vi "LWXPS_PositionerCompensationPreFeedForwardPhaseCorrectionFilterSet.vi"(0 "Positioner Name":string, 1 "XPS Reference IN":refnum<k24>, 5 "Filter Number":i32, 7 "Numerator Frequency":dbl, 9 "Denominator Frequency":dbl, 11 "Phase Correction Gain":dbl, 12 "LabVIEW error IN":errorcluster) -> (4 "XPS Reference OUT":refnum<k24>, 6 "Returned error code":i32, 8 "XPS Error String":string, 15 "LabVIEW error OUT":errorcluster)   [LabVIEW 2014]
uses:
  D:/XPSQ8_LabView_Library/Development/Source/Dll/Newport.XPS.CommandInterface.dll
  Dll/Newport.XPS.CommandInterface.dll
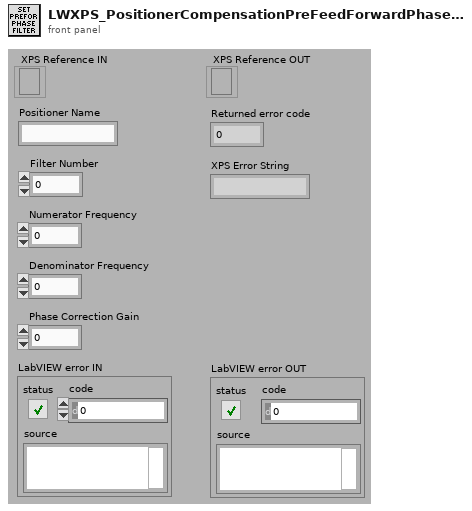
[diagram p1: front panel]
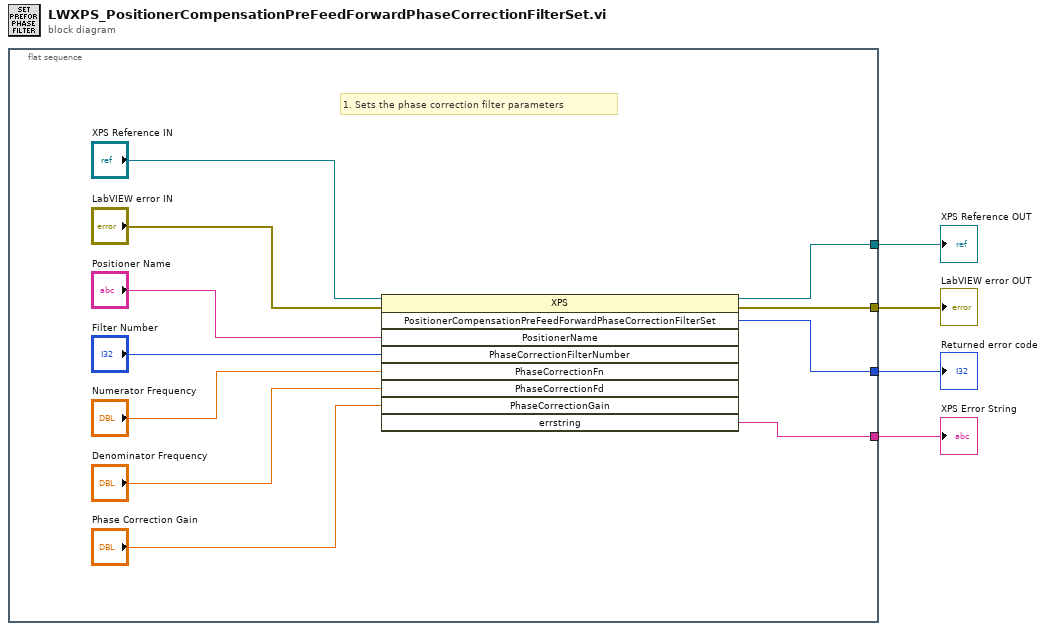
[diagram p0: block diagram]
diagram:
  n1 = flat-sequence {
    tunnel: [w11] -> w4
    tunnel: [w10] -> w3
    tunnel: [w12] -> w2
    tunnel: [w8] -> w1
    frame #0 {
      # "1. Sets the phase correction filter parameters"
      n2 = invoke class="XPS" method="PositionerCompensationPreFeedForwardPhaseCorrectionFilterSet"(reference="XPS Reference IN", error in="LabVIEW error IN", "PositionerName"="Positioner Name", "PhaseCorrectionFilterNumber"="Filter Number", "PhaseCorrectionFn"="Numerator Frequency", "PhaseCorrectionFd"="Denominator Frequency", "PhaseCorrectionGain"="Phase Correction Gain") -> (reference out=w11:refnum<k24>, error out=w10:errorcluster, "PositionerCompensationPreFeedForwardPhaseCorrectionFilterSet"=w12:i32, "errstring"=w8:string)  [unwired: 2 in, 5 out]
    }
  }
  "XPS Error String" <- w1
  "XPS Reference OUT" <- w4
  "LabVIEW error OUT" <- w3
  "Returned error code" <- w2
